vi "reconster.vi"() -> ()   [LabVIEW 2020]
uses:
  <userlib>/_OpenG.lib/array/array.llb/Remove Duplicates from 1D Array (DBL)__ogtk.vi
panel:
  in  "Sorted Array out 2":i32[][](array[numeric])
  out "subarray":i32[](array[numeric])
  in  "Cluster Names":string[](array[string])
  in  "Array 5":variant[](array[variant])
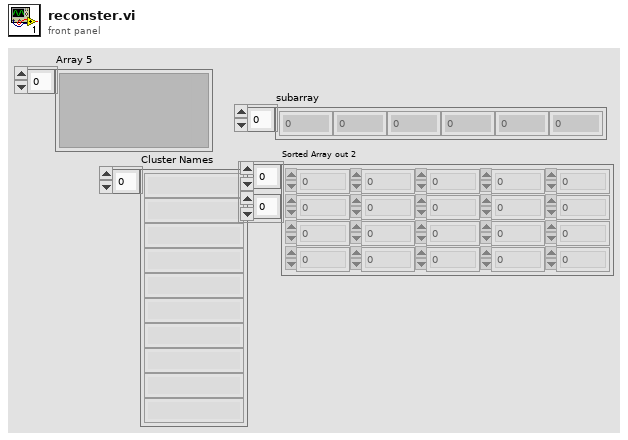
[diagram p1: front panel]
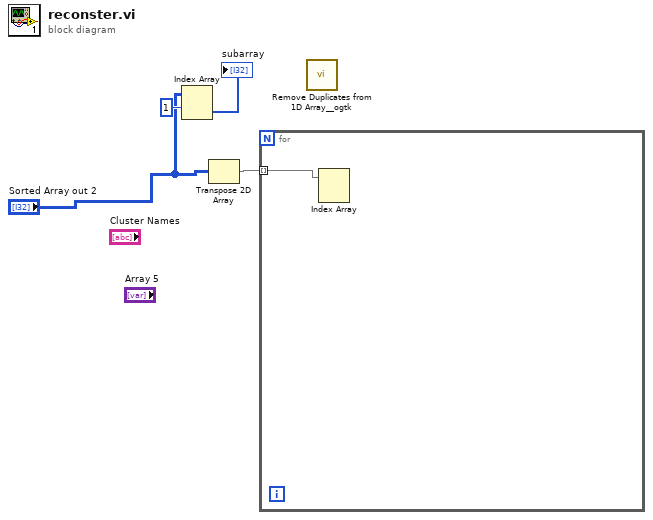
[diagram p0: block diagram]
diagram:
  n1 = Index Array(array="Sorted Array out 2", index (row)=1) -> (element=→"subarray":i32[])  [unwired: 1 in]
  n2 = Transpose 2D Array(2D array="Sorted Array out 2") -> (transposed array=w4:i32[][])
  n3 = for {
    tunnel: w4 -> [w5] mode=indexing
    n4 = Index Array(array=w5) -> ()  [unwired: 2 in, 2 out]
  }
  n5 = call-poly <userlib>:"Remove Duplicates from 1D Array__ogtk.vi"() -> ()  [unwired: 1 in, 2 out]
